vi "TurnToTarget.vi"() -> (3 "On Target":bool)   [LabVIEW 2011]
uses:
  Robot Global Data.vi
panel:
  in  "Timeout":u32=2000
  in  "On Target Threshold":dbl=0.1
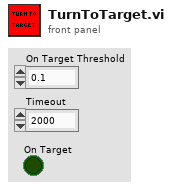
[diagram p1: front panel]
types:
  T1 = typedef "Position Typedef.ctl" = cluster{"X":dbl, "Y":dbl, "Heading":dbl}
  T2 = typedef "Target Typedef.ctl" = cluster{"X":dbl, "Y":dbl, "Deltax":dbl, "Distance":dbl}
  T3 = typedef "CAN Data.ctl" = cluster{"Turret Position":dbl}
  T4 = typedef "WPI_MotorControlDeviceRef.ctl" = cluster{"DeviceStatus":errorcluster, "Type":enum16{"PWM", "CAN"}, "PWM":cluster{"Digital Module":T5, "PWM Channel":T6, "DeadBand":T7}, "CAN":cluster{"Device Number":u8, "Control Mode":T8, "Semaphore":T9, "Max Vout":dbl}, "Invert":bool, "TransformRef":T10, "InvTransformRef":T10}
  T5 = typedef "FPGA_TypedefDigitalModule.ctl" = enum16{"Digital Module 1", "Digital Module 2"}
  T6 = typedef "FPGA_DIOPWMChannel.ctl" = enum8{"PWM 1", "PWM 2", "PWM 3", "PWM 4", "PWM 5", "PWM 6", "PWM 7", "PWM 8", "PWM 9", "PWM 10", "Invalid"}
  T7 = typedef "WPI_PWMDeadband.ctl" = cluster{"Name":string, "maxPositivePwm":i32, "minPositivePwm":i32, "centerPwm":i32, "maxNegativePwm":i32, "minNegativePwm":i32, "angularRange":u16}
  T8 = typedef "WPI_CANJaguar_ControlMode.ctl" = enum8{"Percent VBus", "Current", "Speed", "Position", "Voltage"}
  T9 = typedef "Semaphore RefNum" = refnum<k1>
  T10 = typedef "WPI_PWMTransform_ConPane.ctl" = refnum<vi>
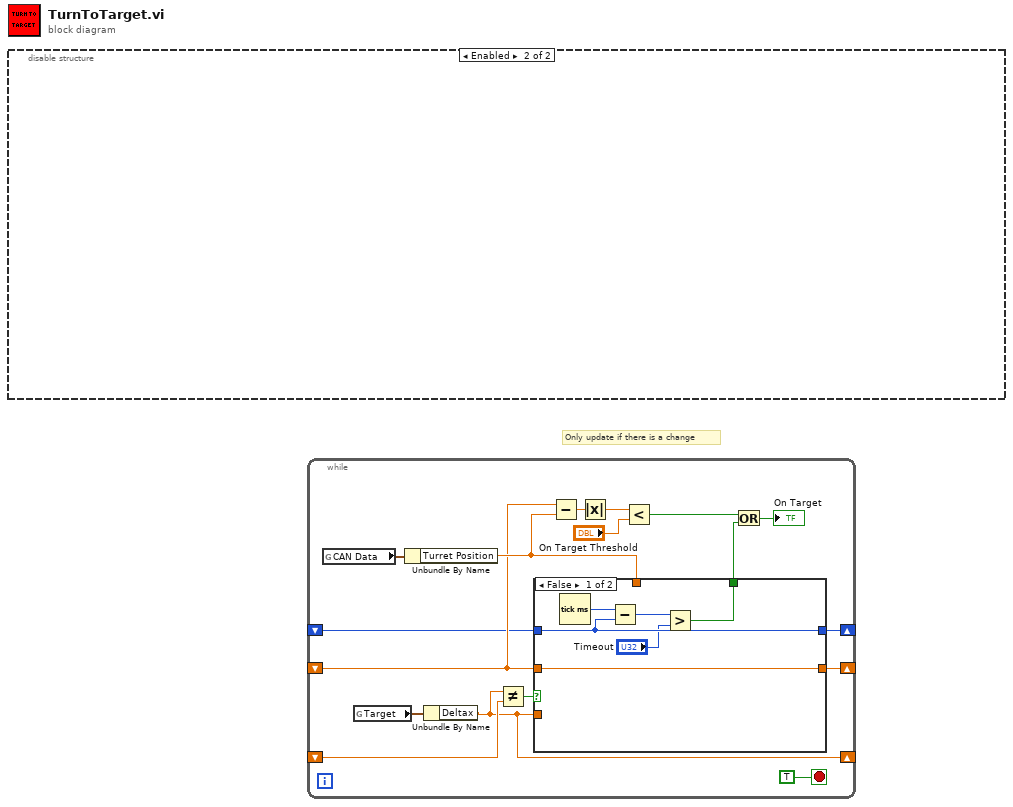
[diagram p0: block diagram]
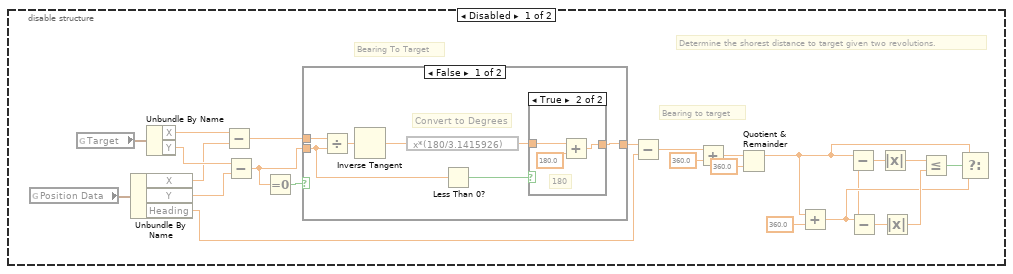
[diagram p2: hidden frame]
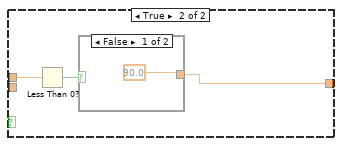
[diagram p4: hidden frame]
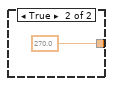
[diagram p5: hidden frame]
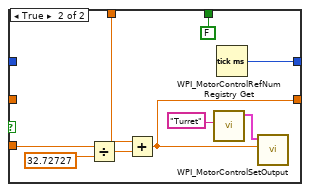
[diagram p6: hidden frame]
diagram:
  # "Only update if there is a change"
  n1 = disable-structure shown="Enabled" {
    frame Disabled {
      # "Bearing to target"
      # "Bearing To Target"
      # "Determine the shorest distance to target given two revolutions."
      n2 = global read "Robot Global Data.vi" "Position Data"() -> (w16:T1)
      n3 = global read "Robot Global Data.vi" "Target"() -> (w17:T2)
      n4 = Unbundle By Name(w16) -> ("X"=w9:dbl, "Y"=w8:dbl, "Heading"=w7:dbl)
      n5 = Unbundle By Name(w17) -> ("X"=w11:dbl, "Y"=w10:dbl)
      n6 = Subtract(x=w11, y=w9) -> (x-y=w13:dbl)
      n7 = Subtract(x=w10, y=w8) -> (x-y=w12:dbl)
      n8 = Equal To 0?(x=w12) -> (x = 0?=w15:bool)
      n9 = case shown="False" w15 {
        tunnel: w13 -> [w31 w37]
        tunnel: [w26 w36] -> w14
        tunnel: w12 -> [w28 _]
        frame False {
          # "Convert to Degrees"
          n10 = Divide(x=w31, y=w28) -> (x/y=w29:dbl)
          n11 = Inverse Tangent(1:w29) -> (0:w30:dbl)
          n12 = expression code="x*(180/3.1415926)"(w30) -> (w25:dbl)
          n13 = Less Than 0?(x=w28) -> (x < 0?=w27:bool)
          n14 = case shown="True" w27 {
            tunnel: [w32 w35] -> w26
            tunnel: w25 -> [w32 w34]
            frame False {
            }
            frame True {
              # "180"
              n15 = Add(x=w34, y=180.0) -> (x+y=w35:dbl)
            }
          }
        }
        frame True {
          n16 = Less Than 0?(x=w37) -> (x < 0?=w38:bool)
          n17 = case shown="False" w38 {
            tunnel: [90.0 ("y") 270.0 ("y")] -> w36
            frame False {
            }
            frame True {
            }
          }
        }
      }
      n18 = Subtract(x=w14, y=w7) -> (x-y=w6:dbl)
      n19 = Add(x=w6, y=360.0) -> (x+y=w4:dbl)
      n20 = Quotient & Remainder(x=w4, y=360.0) -> (x-y*floor(x/y)=w5:dbl)  [unwired: 1 out]
      n21 = Add(x=w5, y=360.0) -> (x+y=w18:dbl)
      n22 = Subtract(x=w18) -> (y=w1:dbl, x-y=w22:dbl)
      n23 = Subtract(x=w5, y=w1) -> (x-y=w23:dbl)
      n24 = Absolute Value(x=w23) -> (abs(x)=w21:dbl)
      n25 = Absolute Value(x=w22) -> (abs(x)=w20:dbl)
      n26 = Less Or Equal?(x=w21, y=w20) -> (x <= y?=w19:bool)
      n27 = Select(t=w5, s=w19, f=w18) -> ()  [unwired: 1 out]
    }
    frame Enabled {
    }
  }
  n28 = while {
    shift-right: [w51] -> _
    shift-left: _ -> [w55]
    shift-right: [w54] -> _
    shift-left: _ -> [w46]
    shift-right: [w45] -> _
    shift-left: _ -> [w44]
    stop <- TRUE stop-if-true
    n29 = global read "Robot Global Data.vi" "CAN Data"() -> (w53:T3)
    n30 = global read "Robot Global Data.vi" "Target"() -> (w52:T2)
    n31 = Unbundle By Name(w53) -> ("Turret Position"=w47:dbl)
    n32 = Unbundle By Name(w52) -> ("Deltax"=w51:dbl)
    n33 = Not Equal?(x=w51, y=w55) -> (x != y?=w56:bool)
    n34 = case shown="False" w56 {
      tunnel: w51 -> [_ w66]
      tunnel: w47 -> [_ w70]
      tunnel: [w63 w69] -> w54
      tunnel: w46 -> [w63 _]
      tunnel: [w61 w65] -> w45
      tunnel: w44 -> [w61 _]
      tunnel: [w58 FALSE] -> w43
      frame False {
        n35 = Tick Count (ms)() -> (millisecond timer value=w62:u32)
        n36 = Subtract(x=w62, y=w61) -> (x-y=w60:u32)
        n37 = Greater?(x=w60, y="Timeout") -> (0:w58:bool)
      }
      frame True {
        n38 = Divide(x=w66, y=32.72727) -> (x/y=w67:dbl)
        n39 = Add(x=w70, y=w67) -> (x+y=w69:dbl)
        n40 = call <vilib>:"WPI_MotorControlRefNum Registry Get.vi"("refnum name"="Turret") -> ("MotorControlDevRef"=w72:T4)  [unwired: 9 in, 1 out]
        n41 = Tick Count (ms)() -> (millisecond timer value=w65:u32)
        n42 = call <vilib>:"WPI_MotorControlSetOutput.vi"("Output"=w69, "MotorControlDevRef"=w72) -> ()  [unwired: 8 in, 2 out]
      }
    }
    n43 = Subtract(x=w46, y=w47) -> (x-y=w48:dbl)
    n44 = Absolute Value(x=w48) -> (abs(x)=w49:dbl)
    n45 = Less?(x=w49, y="On Target Threshold") -> (x < y?=w41:bool)
    n46 = Or(x=w41, y=w43) -> (x .or. y?=→"On Target":bool)
  }
